vi "VNA_Set_Freq.vi"(0 "VISA in":refnum<visa-resource-name>, 1 "Start":dbl, 2 "Stop":dbl, 3 "error in (no error)":errorcluster, 4 "Points":i32) -> (5 "VISA out":refnum<visa-resource-name>, 6 "error out":errorcluster)   [LabVIEW 2017]
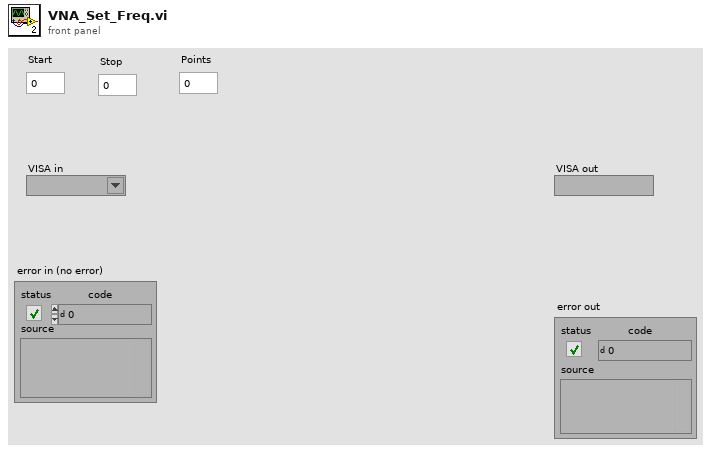
[diagram p1: front panel]
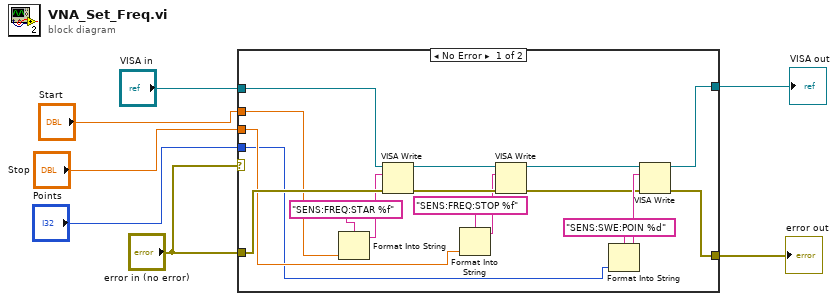
[diagram p0: block diagram]
diagram:
  n1 = case shown="No Error" "error in (no error)" {
    tunnel: "error in (no error)" -> [w24 w26]
    tunnel: [w13 w26] -> w6
    tunnel: [w14 w25] -> w5
    tunnel: "VISA in" -> [w22 w25]
    tunnel: "Start" -> [w16 _]
    tunnel: "Stop" -> [w15 _]
    tunnel: "Points" -> [w10 _]
    frame No Error {
      n2 = Format Into String(format string="SENS:FREQ:STAR %f", w16) -> (resulting string=w19:string)  [unwired: 2 in, 1 out]
      n3 = VISA Write(VISA resource name=w22, write buffer=w19, error in (no error)=w24) -> (VISA resource name out=w21:refnum<visa-resource-name>, error out=w23:errorcluster)  [unwired: 1 out]
      n4 = Format Into String(format string="SENS:FREQ:STOP %f", w15) -> (resulting string=w20:string)  [unwired: 2 in, 1 out]
      n5 = VISA Write(VISA resource name=w21, write buffer=w20, error in (no error)=w23) -> (VISA resource name out=w9:refnum<visa-resource-name>, error out=w8:errorcluster)  [unwired: 1 out]
      n6 = Format Into String(format string="SENS:SWE:POIN %d", w10) -> (resulting string=w12:string)  [unwired: 2 in, 1 out]
      n7 = VISA Write(VISA resource name=w9, write buffer=w12, error in (no error)=w8) -> (VISA resource name out=w14:refnum<visa-resource-name>, error out=w13:errorcluster)  [unwired: 1 out]
    }
    frame Error {
    }
  }
  "VISA out" <- w5
  "error out" <- w6
